vi "Hardware-DI-MinSwitchTime.vi"(8 "Piezo Min Switch [s]":sgl=5e-07 format="%#_6p", 9 "Solenoid Min Switch [s]":sgl=2e-06 format="%#_6p", 11 "DCM Reference":refnum<class "DCM - RT.lvclass">) -> ()   [LabVIEW 2016, in "DSI-RT.lvlib"]
uses:
  DSI-RT.lvlib
  <vilib>/Powertrain Controls/Device Drivers/DCM/Rev0/RT/DCM - RT.lvclass
  <vilib>/Powertrain Controls/Device Drivers/DCM/Rev0/RT/DCM - RT.lvclass/DCM - RT.ctl
  <vilib>/Powertrain Controls/Device Drivers/DCM/Rev0/RT/Read FPGA Reference.vi
  <vilib>/Utility/error.llb/Error Cluster From Error Code.vi
  <vilib>/rvi/errors/niLvFpgaAdjustHostInterfaceError.vi
  <vilib>/rvi/interface/nirviReadWriteControl/nirviReadWriteControl.xnode
  NiFpgaLv.dll
  <vilib>/rvi/interface/Simulation/niFpgaSimulationCallBeginRW.vi
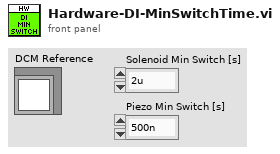
[diagram p1: front panel]
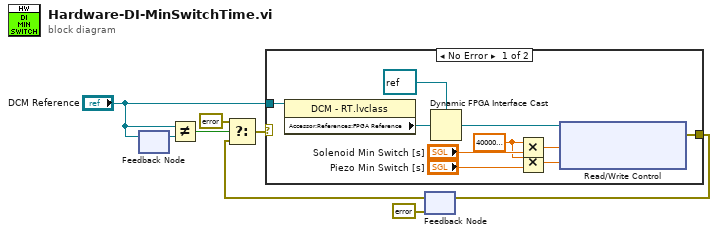
[diagram p0: block diagram]
diagram:
  n1 = feedback #1() -> (w1:refnum<class "DCM - RT.lvclass">)  [unwired: 1 in]
  n2 = feedback-in #1("DCM Reference") -> ()
  n3 = Not Equal?(x="DCM Reference", y=w1) -> (x != y?=w5:bool)
  n4 = feedback #2(errorcluster {"status"=FALSE, "code"=0, "source"=""} ("error IO")) -> (w6:errorcluster)
  n5 = Select(t=errorcluster {"status"=FALSE, "code"=0, "source"=""} ("error out"), s=w5, f=w6) -> (s? t:f=w7:errorcluster)
  n6 = case shown="No Error" w7 {
    selector: w7 -> [_ w19]
    tunnel: "DCM Reference" -> [w15 _]
    tunnel: [w14 w19] -> w3
    frame No Error {
      w9 = sgl 40000000.0 ("x")
      n7 = property class="DCM - RT.lvclass"(reference=w15) -> ("Accessor:References:FPGA Reference"=w17:refnum<k20>)  [unwired: 1 in, 2 out]
      n8 = Dynamic FPGA Interface Cast(Session In=refnum<k20> refnum ("Type"), Type=w17) -> (Session Out=w16:refnum<k20>)
      n9 = Multiply(x=w9, y="Solenoid Min Switch [s]") -> (x*y=w11:sgl)
      n10 = Multiply(x=w9, y="Piezo Min Switch [s]") -> (x*y=w10:sgl)
      n11 = xnode ("Read/Write Control")("FPGA VI Reference In"=w16, "Solenoid Min Switch"=w11, "Piezo Min Switch"=w10) -> ("error out"=w14:errorcluster)  [unwired: 1 in, 1 out]
    }
    frame Error {
    }
  }
  n12 = feedback-in #2(w3) -> ()
